vi "Advance past whitespace and comma.vi"(7 "JSON":string, 9 "Offset":i32, 11 "State in":T1=enum."Leading Whitespace") -> (1 "Offset past match":i32, 3 "State":T1=enum."Value end")   [LabVIEW 2015, in "JSONtext.lvlib"]
uses:
  JSONtext.lvlib
  Parsing State.ctl
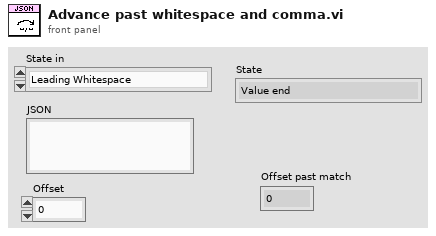
[diagram p1: front panel]
types:
  T1 = typedef "JSONtext.lvlib/Parsing State.ctl" = enum16{"Parser Error", "Object", "Array", "String", "Number/Other", "Leading Whitespace", "Object end", "Array end", "Value end"}
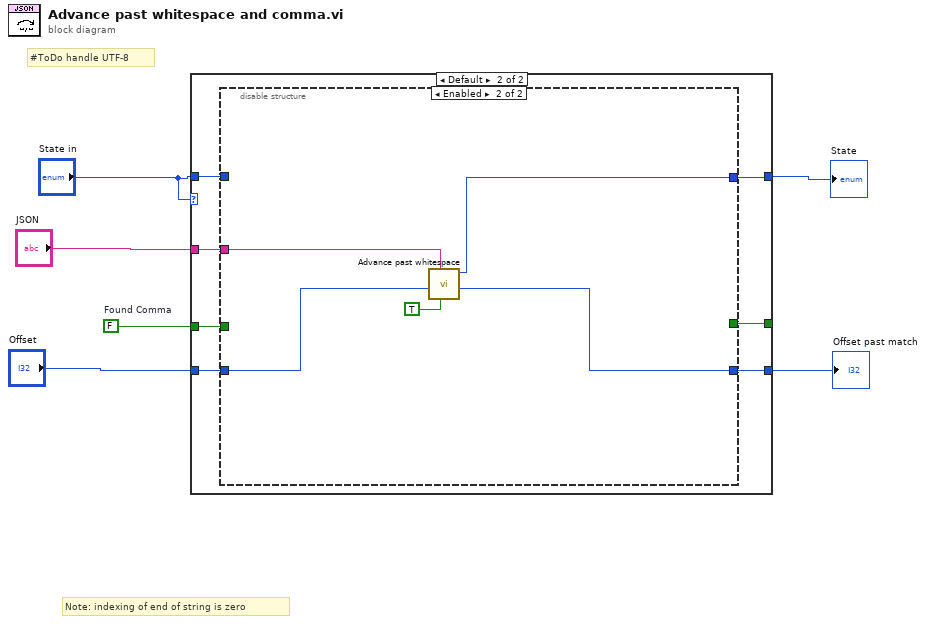
[diagram p0: block diagram]
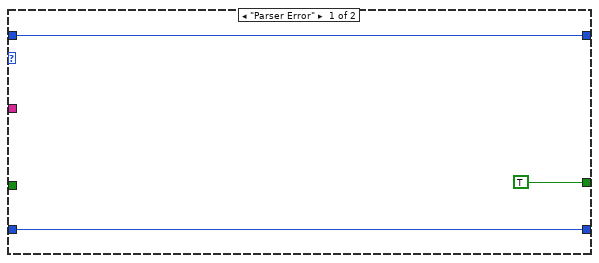
[diagram p2: hidden frame]
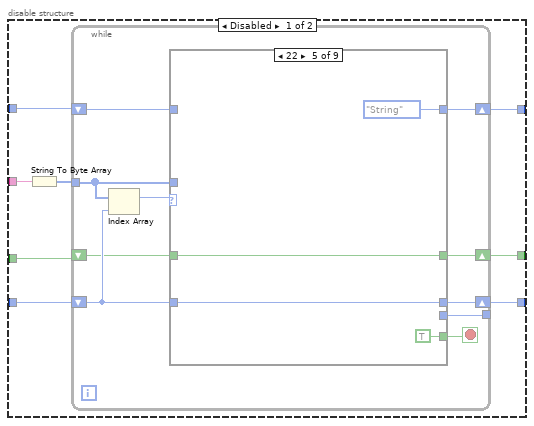
[diagram p3: hidden frame]
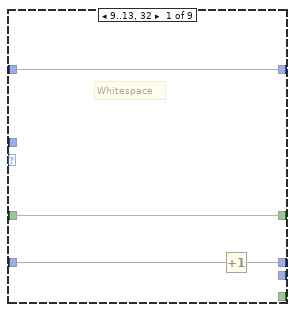
[diagram p4: hidden frame]
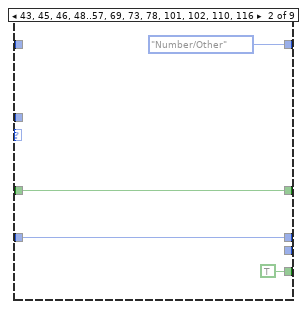
[diagram p5: hidden frame]
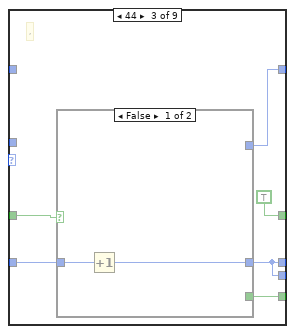
[diagram p6: hidden frame]
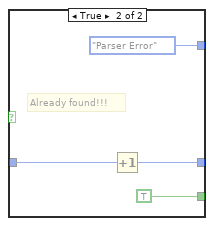
[diagram p7: hidden frame]
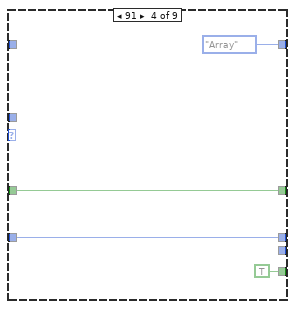
[diagram p8: hidden frame]
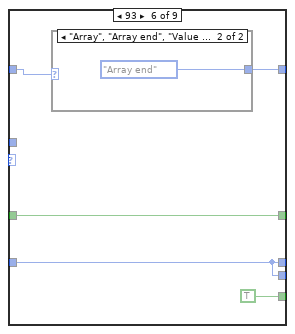
[diagram p9: hidden frame]
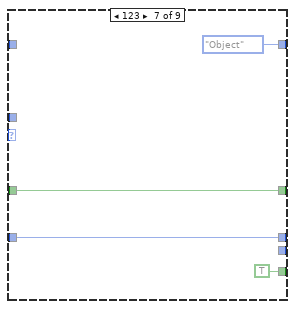
[diagram p11: hidden frame]
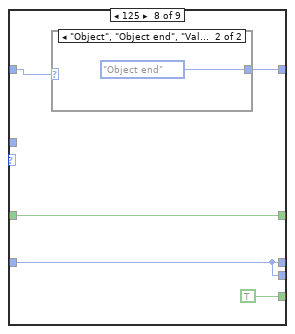
[diagram p12: hidden frame]
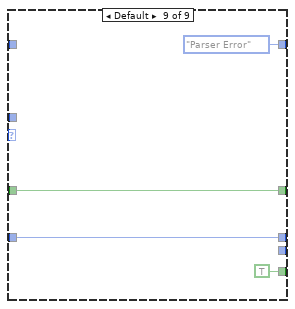
[diagram p14: hidden frame]
diagram:
  w2 = FALSE  # Found Comma
  # "Note: indexing of end of string is zero"
  # "#ToDo handle UTF-8"
  n1 = case shown="Default" "State in" {
    tunnel: [w9 w11] -> w1
    tunnel: [w8 w16] -> w6
    tunnel: "State in" -> [w9 w15]
    tunnel: "Offset" -> [w8 w13]
    tunnel: "JSON" -> [_ w14]
    tunnel: w2 -> [_ w12]
    tunnel: [TRUE ("Found Comma") w10] -> _
    frame "Parser Error" {
    }
    frame Default {
      n2 = disable-structure shown="Enabled" {
        disable-tunnel: [w24 w85] -> w16
        disable-tunnel: w15 -> [w23 _]
        disable-tunnel: w14 -> [w21 w87]
        disable-tunnel: w13 -> [w20 w84]
        disable-tunnel: w12 -> [w19 _]
        disable-tunnel: [w18 w86] -> w11
        disable-tunnel: [w17 _] -> w10
        frame Disabled {
          n3 = String To Byte Array(string=w21) -> (unsigned byte array=w22:u8[])
          n4 = while {
            tunnel: w22 -> [w33]
            shift-right: [w28] -> w24
            shift-left: w20 -> [w29]
            shift-right: [w31] -> w18
            shift-left: w23 -> [w32]
            tunnel: [w27] -> _
            shift-right: [w26] -> w17
            shift-left: w19 -> [w25]
            stop <- w30 stop-if-true
            n5 = Index Array(array=w33, index=w29) -> (element=w34:u8)
            n6 = case shown="22" w34 {
              tunnel: w33 -> [_ _ _ _ _ _ _ _ _]
              tunnel: w32 -> [w38 _ _ _ _ w64 _ w74 _]
              tunnel: [w38 Parsing_State."Number/Other" w43 Parsing_State."Array" Parsing_State."String" w67 Parsing_State."Object" w77 Parsing_State."Parser Error"] -> w31
              tunnel: [_ TRUE w48 TRUE TRUE TRUE TRUE TRUE TRUE] -> w30
              tunnel: w29 -> [w37 w42 w47 w58 w62 w65 w72 w75 w82]
              tunnel: [w36 w42 w46 w58 w62 w65 w72 w75 w82] -> w28
              tunnel: [_ _ w46 _ _ w65 _ w75 _] -> w27
              tunnel: [w35 w41 TRUE w57 w61 w63 w71 w73 w79] -> w26
              tunnel: w25 -> [w35 w41 w45 w57 w61 w63 w71 w73 w79]
              frame 9..13, 32 {
                # "Whitespace"
                n7 = Increment(x=w37) -> (x+1=w36:i32)
              }
              frame 43, 45, 46, 48..57, 69, 73, 78, 101, 102, 110, 116 {
              }
              frame 44 {
                # ","
                n8 = case shown="False" w45 {
                  tunnel: [_ TRUE] -> w48
                  tunnel: w47 -> [w50 w53]
                  tunnel: [w49 w52] -> w46
                  tunnel: [_ Parsing_State."Parser Error"] -> w43
                  frame False {
                    n9 = Increment(x=w50) -> (x+1=w49:i32)
                  }
                  frame True {
                    # "Already found!!!"
                    n10 = Increment(x=w53) -> (x+1=w52:i32)
                  }
                }
              }
              frame 91 {
              }
              frame 34 {
              }
              frame 93 {
                n11 = case shown="\"Array\", \"Array end\", \"Value end\"" w64 {
                  tunnel: [_ Parsing_State."Array end"] -> w67
                  frame Default {
                  }
                  frame "Array", "Array end", "Value end" {
                  }
                }
              }
              frame 123 {
              }
              frame 125 {
                n12 = case shown="\"Object\", \"Object end\", \"Value end\"" w74 {
                  tunnel: [_ Parsing_State."Object end"] -> w77
                  frame Default {
                  }
                  frame "Object", "Object end", "Value end" {
                  }
                }
              }
              frame Default {
              }
            }
          }
        }
        frame Enabled {
          n13 = call "Advance past whitespace.vi"("Past Comma"=TRUE ("Allow Comma"), "JSON"=w87, "Offset"=w84) -> ("Offset of first non-whitespace"=w85:i32, "Parser State"=w86:T1)  [unwired: 7 in]
        }
      }
    }
  }
  "State" <- w1
  "Offset past match" <- w6
